vi "Parse_pyWebscraper_Data.vi"(6 "Row Type":T1, 7 "Column Type":T2, 8 "error in (no error)":errorcluster, 11 "2D Array":string[][](array[string])) -> (0 "error out":errorcluster, 3 "Element":string)   [LabVIEW 2025]
uses:
  Control/Column Type.ctl
  Control/Row Type.ctl
  <vilib>/Utility/error.llb/Error Cluster From Error Code.vi
  <vilib>/ErrorRing/Error Ring.xnode
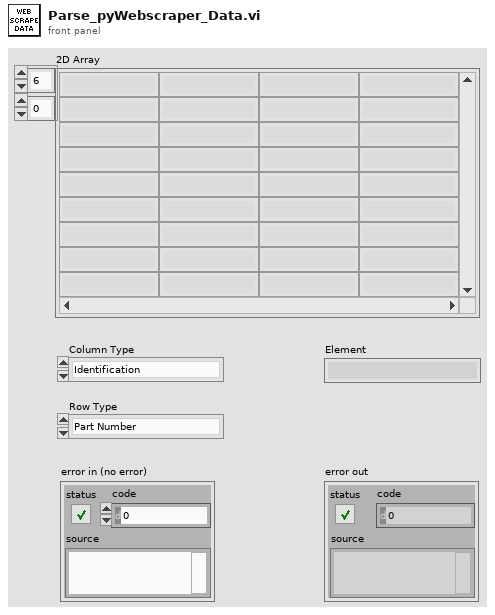
[diagram p1: front panel]
types:
  T1 = typedef "Row Type.ctl" = enum16{"Part Number", "Serial Number", "Model Revision", "Primary FW Rev", "Secondary FW Rev", "Manufacturing Lot Code", "Manufacturer Name", "Manufacturer ID", "Input Voltage", "Output Voltage", "Battery Voltage", "Output Current", "Internal Temperature", "Lifetime Turn On Time", "Turn On Time ", "Event Code", "High Internal Temperature", "Low Battery SOC Alarm", "Low Battery Runtime Alarm", "System Temperature", "User System Name", "User Device Name", "Battery Type"}
  T2 = typedef "Column Type.ctl" = enum16{"Identification", "Description", "Value", "Unit", "Event Code", "Event Start/End", "Threshold", "TimeStamp (Hrs)"}
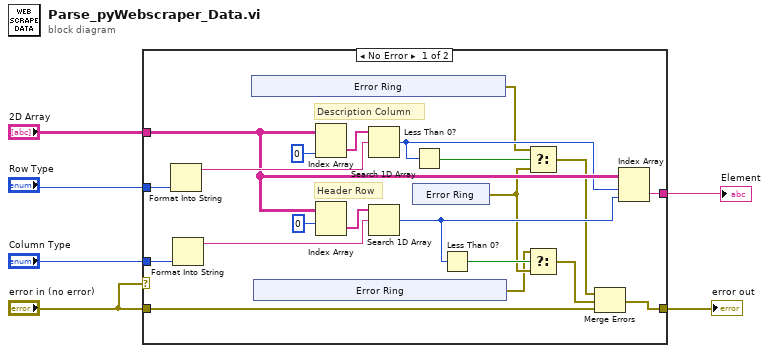
[diagram p0: block diagram]
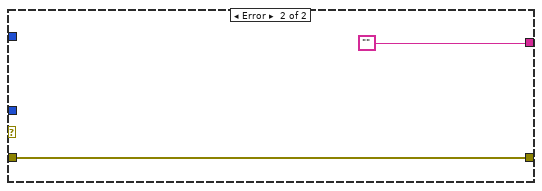
[diagram p2: hidden frame]
diagram:
  n1 = case shown="No Error" "error in (no error)" {
    tunnel: "error in (no error)" -> [w8 w40]
    tunnel: [w7 w40] -> w6
    tunnel: "Row Type" -> [w26 _]
    tunnel: "Column Type" -> [w24 _]
    tunnel: "2D Array" -> [w18 _]
    tunnel: [w19 ""] -> w4
    frame No Error {
      # "Description Column"
      # "Header Row"
      n2 = Format Into String(w26) -> (resulting string=w21:string)  [unwired: 3 in, 1 out]
      n3 = Format Into String(w24) -> (resulting string=w20:string)  [unwired: 3 in, 1 out]
      n4 = xnode "Error Ring"() -> ("error out"=w14:errorcluster)
      n5 = xnode "Error Ring"() -> ("error out"=w11:errorcluster)
      n6 = Index Array(array=w18, index (col)=0 ("disabled index (col)")) -> (element=w22:string[])  [unwired: 1 in]
      n7 = Index Array(array=w18, index (row)=0) -> (element=w23:string[])  [unwired: 1 in]
      n8 = Search 1D Array(1D array=w22, element=w21) -> (index of element=w16:i32)  [unwired: 1 in]
      n9 = Search 1D Array(1D array=w23, element=w20) -> (index of element=w17:i32)  [unwired: 1 in]
      n10 = xnode "Error Ring"() -> ("error out"=w12:errorcluster)
      n11 = Less Than 0?(x=w16) -> (x < 0?=w15:bool)
      n12 = Less Than 0?(x=w17) -> (x < 0?=w13:bool)
      n13 = Select(t=w14, s=w15, f=w12) -> (s? t:f=w10:errorcluster)
      n14 = Select(t=w11, s=w13, f=w12) -> (s? t:f=w9:errorcluster)
      n15 = Merge Errors(w10, w9, w8) -> (w7:errorcluster)
      n16 = Index Array(array=w18, index (row)=w16, index (col)=w17) -> (element=w19:string)
    }
    frame Error {
    }
  }
  "error out" <- w6
  "Element" <- w4
